vi "2283_gyroLogica&Control.vi"(4 "angle rate":dbl, 5 "g input":dbl(knob) scale=-1.0..1.0, 6 "angulo":dbl, 8 "Modificador":bool, 9 "Boton 3":bool, 10 "Boton 2":bool, 11 "Boton 1":bool) -> (2 "g boolean":bool, 3 "angulo deseado":dbl)   [LabVIEW 2014]
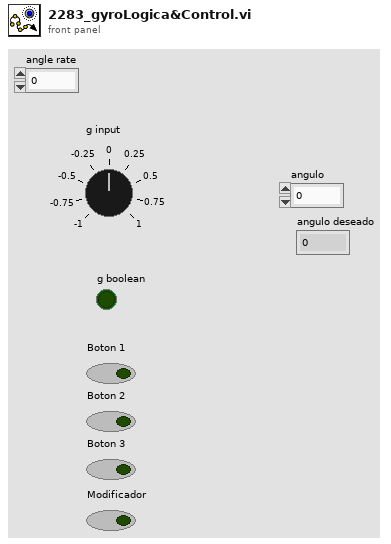
[diagram p1: front panel]
types:
  T1 = enum16{"G Input", "Gyro", "Boton 3 activado", "Boton 2 activado", "Boton 1 activado"}
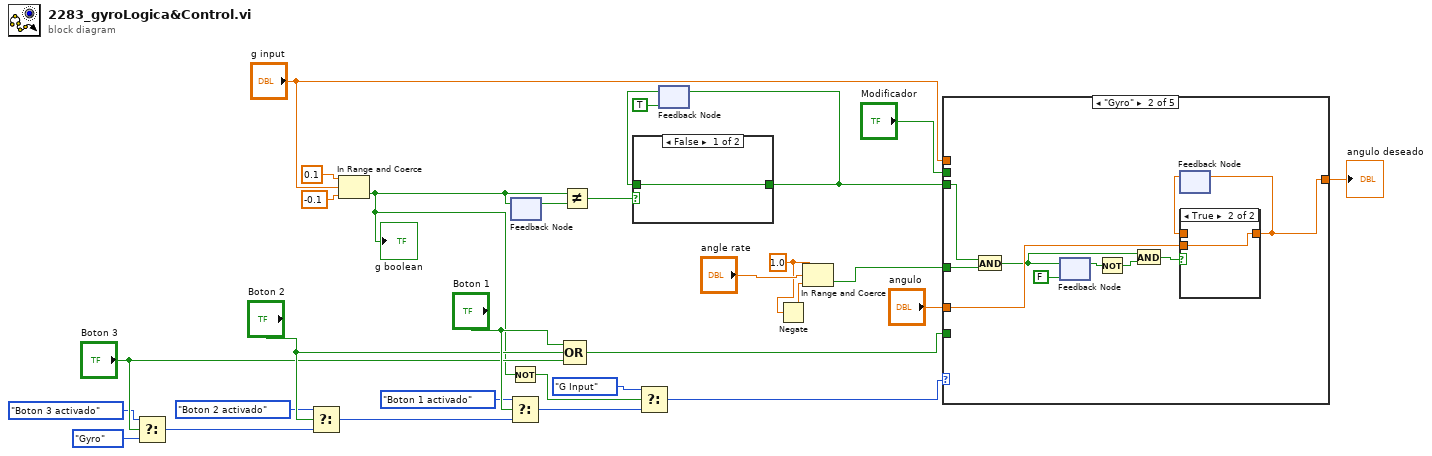
[diagram p0: block diagram]
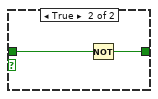
[diagram p2: hidden frame]
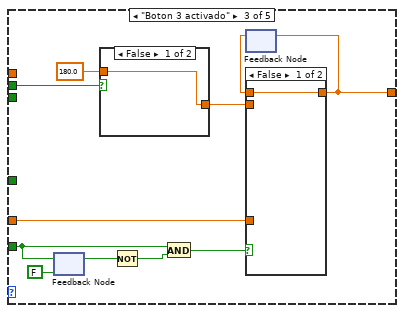
[diagram p5: hidden frame]
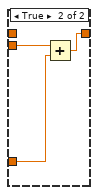
[diagram p6: hidden frame]
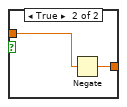
[diagram p7: hidden frame]
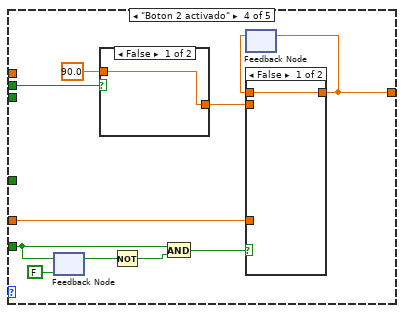
[diagram p8: hidden frame]
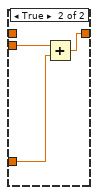
[diagram p9: hidden frame]
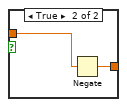
[diagram p10: hidden frame]
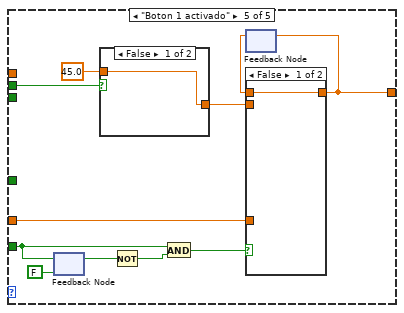
[diagram p11: hidden frame]
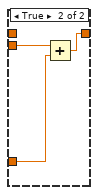
[diagram p12: hidden frame]
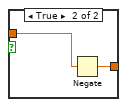
[diagram p13: hidden frame]
diagram:
  w1 = 1.0 ("upper limit")
  n1 = Select(t=T1."Boton 3 activado" ("Enum"), s="Boton 3", f=T1."Gyro" ("Enum")) -> (s? t:f=w28:T1)
  n2 = Select(t=T1."Boton 2 activado" ("Enum"), s="Boton 2", f=w28) -> (s? t:f=w27:T1)
  n3 = In Range and Coerce(upper limit=0.1, x="g input", lower limit=-0.1) -> (In Range?=w5:bool)  [unwired: 1 out]
  "g boolean" <- w5
  n4 = Not(x=w5) -> (.not. x?=w4:bool)
  n5 = Select(t=T1."Boton 1 activado" ("Enum"), s="Boton 1", f=w27) -> (s? t:f=w11:T1)
  n6 = feedback-in #1(w5) -> ()
  n7 = feedback #1() -> (w22:bool)  [unwired: 1 in]
  n8 = Not Equal?(x=w5, y=w22) -> (x != y?=w21:bool)
  n9 = Compound Arithmetic op=OR("Boton 1", "Boton 2", "Boton 3") -> (w12:bool)
  n10 = Select(t=T1."G Input" ("Enum"), s=w4, f=w11) -> (s? t:f=w10:T1)
  n11 = feedback #2(TRUE) -> (w20:bool)
  n12 = case shown="False" w21 {
    tunnel: [w31 w33] -> w18
    tunnel: w20 -> [w31 w32]
    frame False {
    }
    frame True {
      n13 = Not(x=w32) -> (.not. x?=w33:bool)
    }
  }
  n14 = feedback-in #2(w18) -> ()
  n15 = Negate(x=w1) -> (-x=w2:dbl)
  n16 = In Range and Coerce(upper limit=w1, x="angle rate", lower limit=w2) -> (In Range?=w23:bool)  [unwired: 1 out]
  n17 = case shown="\"Gyro\"" w10 {
    tunnel: "angulo" -> [_ w44 w48 w67 w86]
    tunnel: w23 -> [_ w42 _ _ _]
    tunnel: w18 -> [_ w41 _ _ _]
    tunnel: [w34 w35 w47 w65 w83] -> w17
    tunnel: "Modificador" -> [_ _ w50 w68 w93]
    tunnel: w12 -> [_ _ w49 w66 w85]
    tunnel: "g input" -> [w34 _ _ _ _]
    frame "G Input", Default {
    }
    frame "Gyro" {
      n18 = And(x=w41, y=w42) -> (x .and. y?=w38:bool)
      n19 = feedback #3(FALSE) -> (w39:bool)
      n20 = feedback-in #3(w38) -> ()
      n21 = Not(x=w39) -> (.not. x?=w40:bool)
      n22 = And(x=w38, y=w40) -> (x .and. y?=w37:bool)
      n23 = feedback #4() -> (w43:dbl)  [unwired: 1 in]
      n24 = case shown="True" w37 {
        tunnel: w44 -> [_ w46]
        tunnel: [w45 w46] -> w35
        tunnel: w43 -> [w45 _]
        frame False {
        }
        frame True {
        }
      }
      n25 = feedback-in #4(w35) -> ()
    }
    frame "Boton 3 activado" {
      n26 = feedback #5(FALSE) -> (w53:bool)
      n27 = feedback-in #5(w49) -> ()
      n28 = case shown="False" w50 {
        tunnel: 180.0 ("angulo") -> [w62 w64]
        tunnel: [w62 w63] -> w56
        frame False {
        }
        frame True {
          n29 = Negate(x=w64) -> (-x=w63:dbl)
        }
      }
      n30 = Not(x=w53) -> (.not. x?=w54:bool)
      n31 = And(x=w49, y=w54) -> (x .and. y?=w55:bool)
      n32 = feedback #6() -> (w57:dbl)  [unwired: 1 in]
      n33 = case shown="False" w55 {
        tunnel: w56 -> [_ w61]
        tunnel: w48 -> [_ w60]
        tunnel: [w58 w59] -> w47
        tunnel: w57 -> [w58 _]
        frame False {
        }
        frame True {
          n34 = Add(x=w61, y=w60) -> (x+y=w59:dbl)
        }
      }
      n35 = feedback-in #6(w47) -> ()
    }
    frame "Boton 2 activado" {
      n36 = feedback #7(FALSE) -> (w71:bool)
      n37 = feedback-in #7(w66) -> ()
      n38 = case shown="False" w68 {
        tunnel: 90.0 ("angulo") -> [w80 w82]
        tunnel: [w80 w81] -> w74
        frame False {
        }
        frame True {
          n39 = Negate(x=w82) -> (-x=w81:dbl)
        }
      }
      n40 = Not(x=w71) -> (.not. x?=w72:bool)
      n41 = And(x=w66, y=w72) -> (x .and. y?=w73:bool)
      n42 = feedback #8() -> (w75:dbl)  [unwired: 1 in]
      n43 = case shown="False" w73 {
        tunnel: w74 -> [_ w79]
        tunnel: w67 -> [_ w78]
        tunnel: [w76 w77] -> w65
        tunnel: w75 -> [w76 _]
        frame False {
        }
        frame True {
          n44 = Add(x=w79, y=w78) -> (x+y=w77:dbl)
        }
      }
      n45 = feedback-in #8(w65) -> ()
    }
    frame "Boton 1 activado" {
      n46 = feedback #9(FALSE) -> (w90:bool)
      n47 = feedback-in #9(w85) -> ()
      n48 = case shown="False" w93 {
        tunnel: 45.0 ("angulo") -> [w98 w100]
        tunnel: [w98 w99] -> w87
        frame False {
        }
        frame True {
          n49 = Negate(x=w100) -> (-x=w99:dbl)
        }
      }
      n50 = Not(x=w90) -> (.not. x?=w89:bool)
      n51 = And(x=w85, y=w89) -> (x .and. y?=w88:bool)
      n52 = feedback #10() -> (w84:dbl)  [unwired: 1 in]
      n53 = case shown="False" w88 {
        tunnel: w87 -> [_ w97]
        tunnel: w86 -> [_ w96]
        tunnel: [w94 w95] -> w83
        tunnel: w84 -> [w94 _]
        frame False {
        }
        frame True {
          n54 = Add(x=w97, y=w96) -> (x+y=w95:dbl)
        }
      }
      n55 = feedback-in #10(w83) -> ()
    }
  }
  "angulo deseado" <- w17
